vi "07_Project_5_Temp_Measure.vi"() -> ()   [LabVIEW 2014]
panel:
  out "Temperature History":dbl(graph)
  out "Current Temperature":dbl
  in  "stop (F)":bool
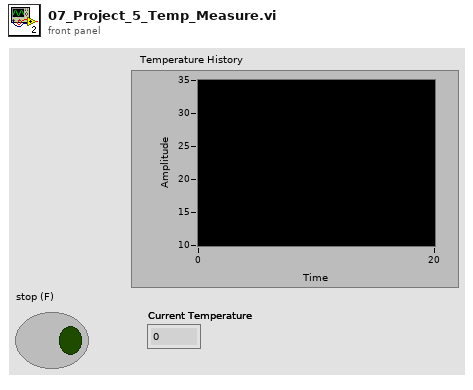
[diagram p1: front panel]
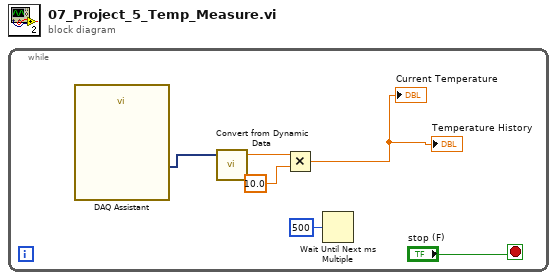
[diagram p0: block diagram]
diagram:
  n1 = while {
    stop <- "stop (F)" stop-if-true
    n2 = call "DAQ Assistant"() -> ("data"=w4:dynamicdata)  [unwired: 16 in, 3 out]
    n3 = call "Convert from Dynamic Data"("Dynamic Data Type"=w4) -> ("Scalar"=w2:dbl)  [unwired: 3 in]
    n4 = Multiply(x=w2, y=10.0) -> (x*y=→"Current Temperature" →"Temperature History":dbl)
    n5 = Wait Until Next ms Multiple(millisecond multiple=u32 500) -> ()  [unwired: 1 out]
  }
